vi "To Pythonic - Float Array.vi"(3 "Precision (6)":i16, 4 "Float Array":dbl[](array[numeric])) -> (1 "Pythonic Value":string)   [LabVIEW 2016, in "OPI.lvclass"]
doc: "Convert LabVIEW data into valid pythonic representation."
uses:
  OPI.lvclass
  <vilib>/AdvancedString/Join Strings.vi
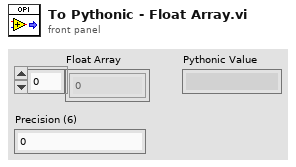
[diagram p1: front panel]
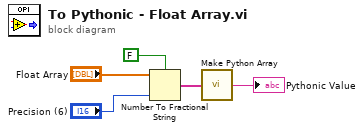
[diagram p0: block diagram]
diagram:
  n1 = Number To Fractional String(use system decimal point (T)=FALSE, number="Float Array", precision (6)="Precision (6)") -> (F-format string=w1:string[])  [unwired: 1 in]
  n2 = call "Make Python Array.vi"("Pythonic Values"=w1) -> ("Pythonic Array"=→"Pythonic Value":string)
